vi "Periodic Tasks.vi"   [LabVIEW 2011]
doc: "This VI runs in parallel to other tasks. It can contain as many user-defined periodic loops as you need. These can carry out PID or other sorts of timed response."
uses:
  <vilib>/Rock Robotics/SystemInterfaces/Utilities/FPGA_UtilitiesLED State.ctl
  <vilib>/Rock Robotics/SystemInterfaces/Utilities/FPGA_UtilitiesLED Source.ctl
  <vilib>/Rock Robotics/WPI/Relay/WPI_RelayValue.ctl
  System Set Points and States.vi
  Robot Global Data.vi
  <vilib>/Rock Robotics/WPI/Compressor/WPI_CompressorGetSetRefNum.vi
types:
  T1 = typedef "FPGA_UtilitiesLED State.ctl" = enum16{"Off", "On", "Toggle"}
  T2 = typedef "FPGA_UtilitiesLED Source.ctl" = enum16{"User LED", "FPGA LED"}
  T3 = typedef "WPI_CompressorDevRef.ctl" = cluster{"DevStatus":errorcluster, "DigitalInputDevRef":T4, "RelayDevRef":T7}
  T4 = typedef "WPI_DigitalInputDevRef.ctl" = cluster{"DevStatus":errorcluster, "DIO Channel":T5, "Digital Module":T6}
  T5 = typedef "FPGA_DIOChannel.ctl" = enum8{"DIO 1", "DIO 2", "DIO 3", "DIO 4", "DIO 5", "DIO 6", "DIO 7", "DIO 8", "DIO 9", "DIO 10", "DIO 11", "DIO 12", "DIO 13", "DIO 14", "Invalid"}
  T6 = typedef "FPGA_TypedefDigitalModule.ctl" = enum16{"Digital Module 1", "Digital Module 2"}
  T7 = typedef "WPI_RelayDevRef.ctl" = cluster{"DevStatus":errorcluster, "Relay Channel":T8, "Digital Module":T6, "Relay Direction":T9}
  T8 = typedef "FPGA_DIORelayChannel.ctl" = enum8{"Relay 1", "Relay 2", "Relay 3", "Relay 4", "Relay 5", "Relay 6", "Relay 7", "Relay 8", "Invalid"}
  T9 = typedef "WPI_RelayDirection.ctl" = enum16{"Both directions", "Forward only", "Reverse only"}
  T10 = typedef "WPI_RelayValue.ctl" = enum16{"Off", "On", "Forward", "Reverse"}
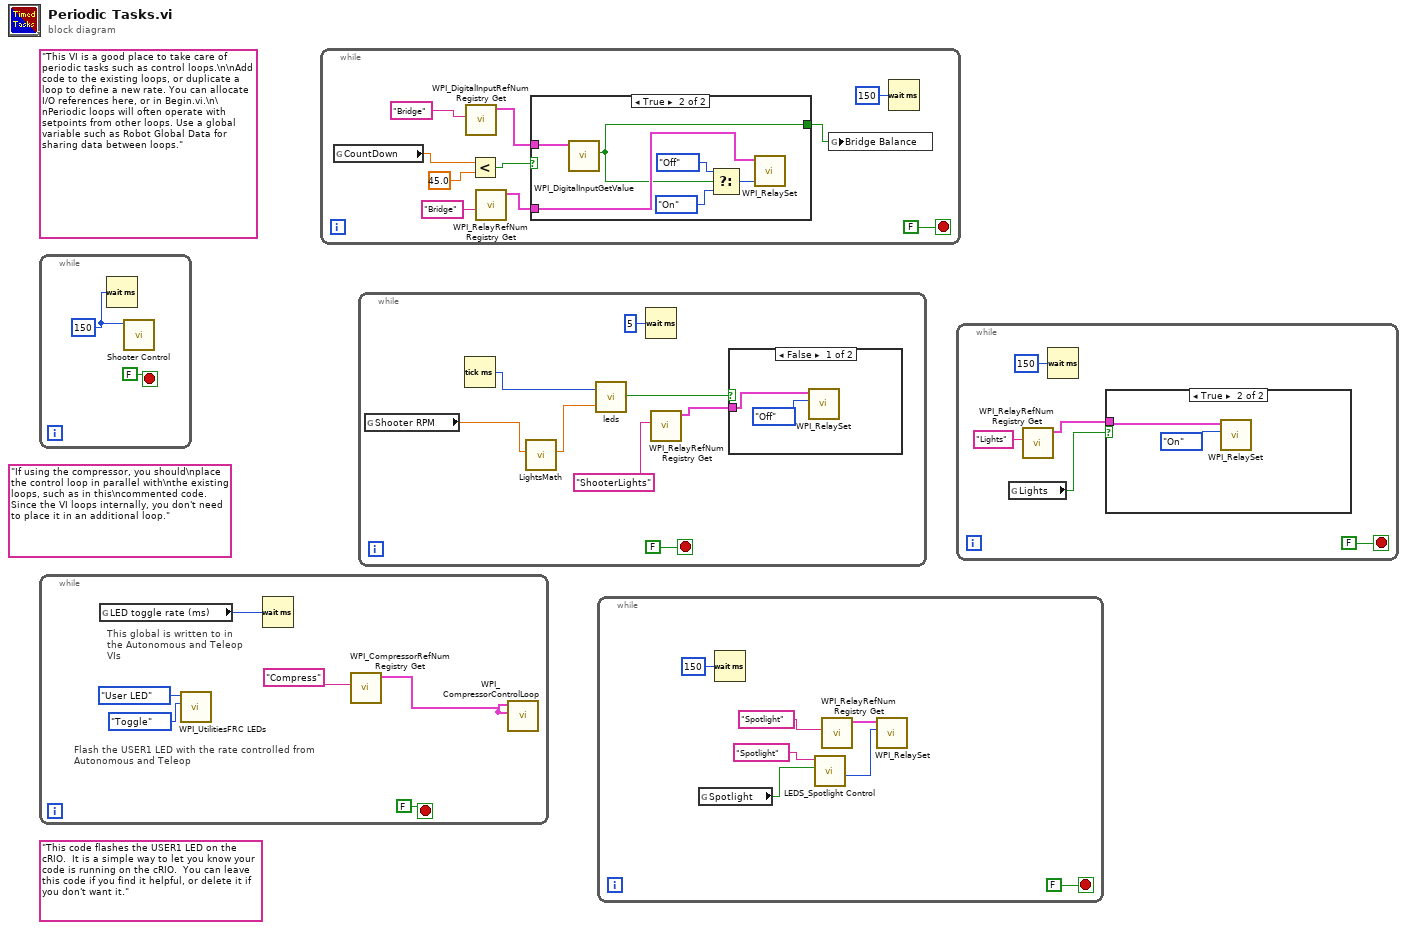
[diagram p0: block diagram]
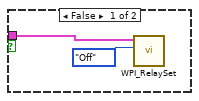
[diagram p2: hidden frame]
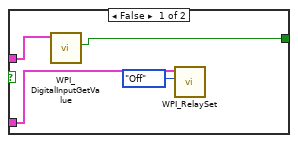
[diagram p3: hidden frame]
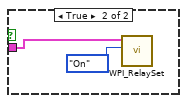
[diagram p4: hidden frame]
diagram:
  (unwired) "If using the compressor, you should\nplace the control loop in parallel with\nthe existing loops, such as in this\ncommented code. Since the VI loops internally, you don't need to place it in an additional loop."
  (unwired) "This code flashes the USER1 LED on the cRIO.  It is a simple way to let you know your code is running on the cRIO.  You can leave this code if you find it helpful, or delete it if you don't want it."
  (unwired) "This VI is a good place to take care of periodic tasks such as control loops.\n\nAdd code to the existing loops, or duplicate a loop to define a new rate. You can allocate I/O references here, or in Begin.vi.\n\nPeriodic loops will often operate with setpoints from other loops. Use a global variable such as Robot Global Data for sharing data between loops."
  n1 = while {
    stop <- FALSE stop-if-true
    w1 = u32 150 ("milliseconds to wait")
    n2 = Wait (ms)(milliseconds to wait=w1) -> ()  [unwired: 1 out]
    n3 = call "Shooter Control.vi"("Time Delay Milli"=w1) -> ()  [unwired: 11 in]
  }
  n4 = while {
    stop <- FALSE stop-if-true
    # "This global is written to in the Autonomous and Teleop VIs"
    # "Flash the USER1 LED with the rate controlled from Autonomous and Teleop"
    n5 = global read "Robot Global Data.vi" "LED toggle rate (ms)"() -> (w5:u32)
    n6 = call <vilib>:"WPI_UtilitiesFRC LEDs.vi"("State"=FPGA_UtilitiesLED_State."Toggle", "LED Type"=FPGA_UtilitiesLED_Source."User LED") -> ()  [unwired: 1 in, 9 out]
    n7 = Wait (ms)(milliseconds to wait=w5) -> ()  [unwired: 1 out]
    n8 = call <vilib>:"WPI_CompressorRefNum Registry Get.vi"("refnum name"="Compress") -> ("CompressorDevRef"=w3:T3)  [unwired: 9 in, 1 out]
    n9 = call <vilib>:"WPI_CompressorControlLoop.vi"("CompressorDevRef 2"=w3, "CompressorDevRef"=w3) -> ()  [unwired: 10 in]
  }
  n10 = while {
    stop <- FALSE stop-if-true
    n11 = global read "System Set Points and States.vi" "CountDown"() -> (w11:dbl)
    n12 = call <vilib>:"WPI_DigitalInputRefNum Registry Get.vi"("refnum name"="Bridge") -> ("DigitalInputDevRef"=w18:T4)  [unwired: 9 in, 1 out]
    n13 = Less?(x=w11, y=45.0) -> (x < y?=w16:bool)
    n14 = call <vilib>:"WPI_RelayRefNum Registry Get.vi"("refnum name"="Bridge") -> ("RelayDevRef"=w14:T7)  [unwired: 9 in, 1 out]
    n15 = case shown="True" w16 {
      tunnel: w18 -> [w20 w28]
      tunnel: w14 -> [w22 w24]
      tunnel: [w19 w23] -> w12
      frame False {
        n16 = call <vilib>:"WPI_DigitalInputGetValue.vi"("DigitalInputDevRef"=w20) -> ("Value"=w19:bool)  [unwired: 8 in, 2 out]
        n17 = call <vilib>:"WPI_RelaySet.vi"("RelayValue"=WPI_RelayValue."Off", "RelayDevRef"=w22) -> ()  [unwired: 8 in, 2 out]
      }
      frame True {
        n18 = call <vilib>:"WPI_DigitalInputGetValue.vi"("DigitalInputDevRef"=w28) -> ("Value"=w23:bool)  [unwired: 8 in, 2 out]
        n19 = Select(t=WPI_RelayValue."Off" ("Relay State"), s=w23, f=WPI_RelayValue."On" ("Relay State")) -> (s? t:f=w27:T10)
        n20 = call <vilib>:"WPI_RelaySet.vi"("RelayValue"=w27, "RelayDevRef"=w24) -> ()  [unwired: 8 in, 2 out]
      }
    }
    n21 = global write "System Set Points and States.vi" "Bridge Balance"(w12) -> ()
    n22 = Wait (ms)(milliseconds to wait=u32 150) -> ()  [unwired: 1 out]
  }
  n23 = while {
    stop <- FALSE stop-if-true
    n24 = global read "System Set Points and States.vi" "Shooter RPM"() -> (w33:dbl)
    n25 = Tick Count (ms)() -> (millisecond timer value=w36:u32)
    n26 = call "LightsMath.vi"("Shooter RPM"=w33) -> ("Light Timing"=w32:dbl)  [unwired: 10 in]
    n27 = call "leds.vi"("range (centisec)"=w32, "input"=w36) -> ("Output"=w30:bool)
    n28 = Wait (ms)(milliseconds to wait=u32 5) -> ()  [unwired: 1 out]
    n29 = call <vilib>:"WPI_RelayRefNum Registry Get.vi"("refnum name"="ShooterLights") -> ("RelayDevRef"=w31:T7)  [unwired: 9 in, 1 out]
    n30 = case shown="False" w30 {
      tunnel: w31 -> [w37 w39]
      frame False {
        n31 = call <vilib>:"WPI_RelaySet.vi"("RelayValue"=WPI_RelayValue."Off", "RelayDevRef"=w37) -> ()  [unwired: 8 in, 2 out]
      }
      frame True {
        n32 = call <vilib>:"WPI_RelaySet.vi"("RelayValue"=WPI_RelayValue."On", "RelayDevRef"=w39) -> ()  [unwired: 8 in, 2 out]
      }
    }
  }
  n33 = while {
    stop <- FALSE stop-if-true
    n34 = global read "System Set Points and States.vi" "Spotlight"() -> (w42:bool)
    n35 = Wait (ms)(milliseconds to wait=u32 150) -> ()  [unwired: 1 out]
    n36 = call "LEDS_Spotlight Control.vi"("Name"="Spotlight", "Button"=w42) -> ("Relay State"=w45:T10)  [unwired: 8 in]
    n37 = call <vilib>:"WPI_RelayRefNum Registry Get.vi"("refnum name"="Spotlight") -> ("RelayDevRef"=w47:T7)  [unwired: 9 in, 1 out]
    n38 = call <vilib>:"WPI_RelaySet.vi"("RelayValue"=w45, "RelayDevRef"=w47) -> ()  [unwired: 8 in, 2 out]
  }
  n39 = while {
    stop <- FALSE stop-if-true
    n40 = global read "System Set Points and States.vi" "Lights"() -> (w50:bool)
    n41 = call <vilib>:"WPI_RelayRefNum Registry Get.vi"("refnum name"="Lights") -> ("RelayDevRef"=w52:T7)  [unwired: 9 in, 1 out]
    n42 = Wait (ms)(milliseconds to wait=u32 150) -> ()  [unwired: 1 out]
    n43 = case shown="True" w50 {
      tunnel: w52 -> [w54 w56]
      frame False {
        n44 = call <vilib>:"WPI_RelaySet.vi"("RelayValue"=WPI_RelayValue."Off", "RelayDevRef"=w54) -> ()  [unwired: 8 in, 2 out]
      }
      frame True {
        n45 = call <vilib>:"WPI_RelaySet.vi"("RelayValue"=WPI_RelayValue."On", "RelayDevRef"=w56) -> ()  [unwired: 8 in, 2 out]
      }
    }
  }
